vi "Write Loop runs.vi"(10 "Loop runs":cluster{"Current":u32, "Total":u32}, 11 "Measurements in":refnum<class "Measurement.lvclass">) -> (3 "Measurements out":refnum<class "Measurement.lvclass">)   [LabVIEW 2020, in "Measurement.lvclass"]
uses:
  Measurement.lvclass
  Measurement.lvclass/Measurement.ctl
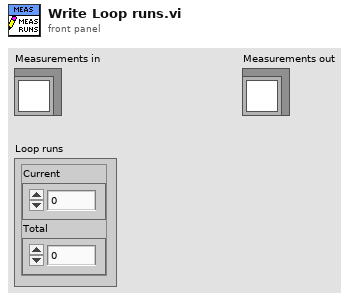
[diagram p1: front panel]
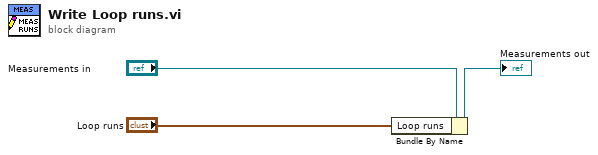
[diagram p0: block diagram]
diagram:
  n1 = Bundle By Name(cluster="Measurements in", "Loop runs"="Loop runs") -> (→"Measurements out":refnum<class "Measurement.lvclass">)
